vi "GetInstVisaHandle.vi"(8 "error in (no error)":errorcluster, 11 "SpecA_MXA in":refnum<class "SpecA_MXA.lvclass">) -> (0 "error out":errorcluster, 2 "VISA resource name out":refnum<visa-resource-name>, 3 "SpecA_MXA out":refnum<class "SpecA_MXA.lvclass">)   [LabVIEW 2014, in "SpecA_MXA.lvclass"]
uses:
  SpecA_MXA.lvclass
  SpecA_MXA.lvclass/SpecA_MXA.ctl
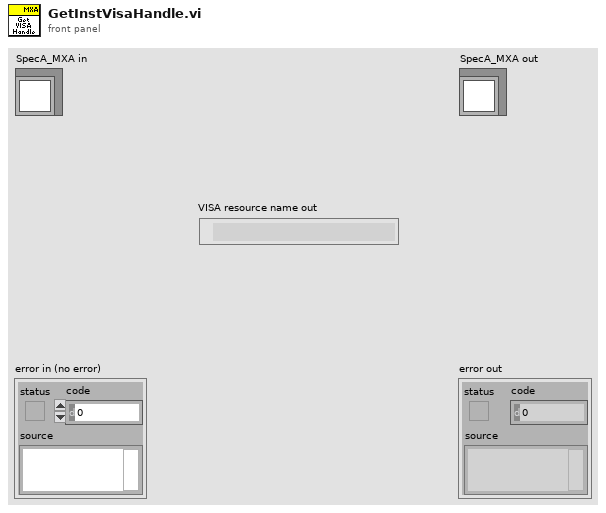
[diagram p1: front panel]
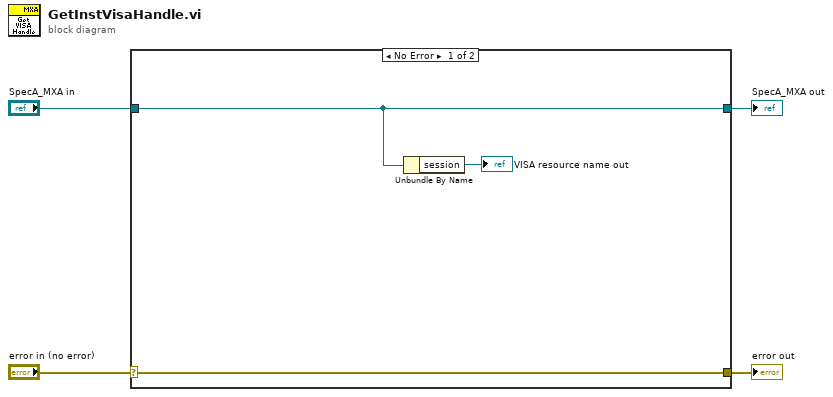
[diagram p0: block diagram]
diagram:
  n1 = case shown="No Error" "error in (no error)" {
    selector: "error in (no error)" -> [w7 w9]
    tunnel: [w7 w9] -> w3
    tunnel: [w6 w8] -> w1
    tunnel: "SpecA_MXA in" -> [w6 w8]
    frame No Error {
      n2 = Unbundle By Name(w6) -> ("session"=→"VISA resource name out":refnum<visa-resource-name>)
    }
    frame Error {
    }
  }
  "error out" <- w3
  "SpecA_MXA out" <- w1
